vi "Tag Metadata Write Tags.vi"(0 "File Path":path, 7 "Tags Group Array":string[][](array[string]), 11 "Error In":errorcluster) -> (15 "Error Out":errorcluster)   [LabVIEW 2020]
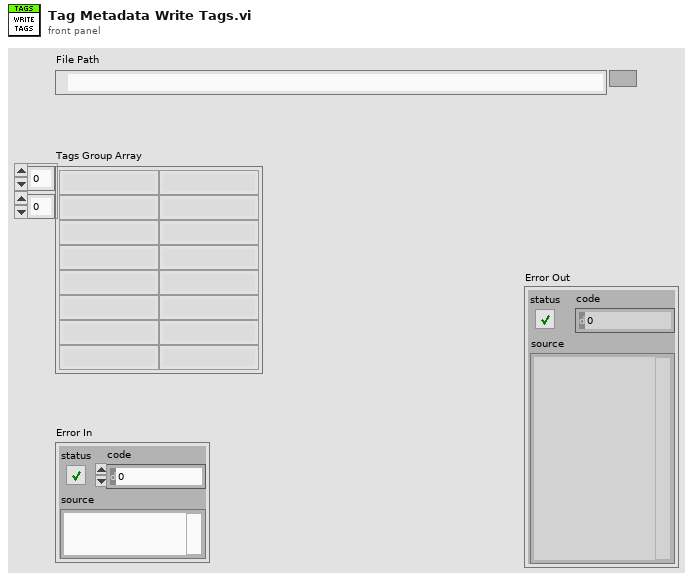
[diagram p1: front panel]
types:
  T1 = enum16{"open", "replace", "create", "open or create", "replace or create", "replace or create with confirmation"}
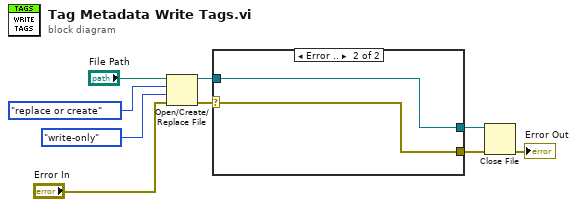
[diagram p0: block diagram]
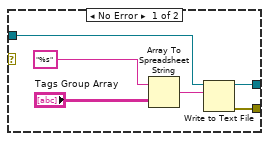
[diagram p2: hidden frame]
diagram:
  n1 = Open/Create/Replace File(file path (use dialog)="File Path", error in="Error In", operation (0:open)=T1."replace or create", access (0:read/write)=enum16{"read/write", "read-only", "write-only"}."write-only") -> (refnum out=w9:refnum<file>, error out=w5:errorcluster)  [unwired: 2 in, 1 out]
  n2 = case shown="Error .." w5 {
    selector: w5 -> [_ w16]
    tunnel: w9 -> [w13 w17]
    tunnel: [w12 w17] -> w4
    tunnel: [w10 w16] -> w3
    frame No Error {
      n3 = Array To Spreadsheet String(array="Tags Group Array", 3:"%s") -> (spreadsheet string=w14:string)  [unwired: 1 in]
      n4 = Write to Text File(file (use dialog)=w13, text=w14) -> (refnum out=w12:refnum<file>, error out=w10:errorcluster)  [unwired: 2 in, 1 out]
    }
    frame Error {
    }
  }
  n5 = Close File(refnum=w4, error in=w3) -> (error out=→"Error Out":errorcluster)  [unwired: 1 out]
